vi "Determine angular axis.vi"(0 "System no.":i32=1 min=1 max=4 step=1, 2 "Axis 1":string, 3 "Axis 2":string, 5 "error in":errorcluster) -> (14 "Ang. axis out":string, 15 "Index of axis\nin Global2":i32, 16 "NC axis 1":string, 17 "NC axis 2":string, 19 "error out":errorcluster)   [LabVIEW 2020]
doc: "Determines angular axis spanned by Axis 1 and Axis 2, and NanoCube axis identifiers corresponding with Axis 1 and Axis 2."
uses:
  General command.llb/Controller names.ctl
  General command.llb/Global2 (Array).vi
panel:
  # "Determines angular axis spanned by Axis 1 and Axis 2, and \nNanoCube axis identifiers corresponding with Axis 1 and Axis 2."
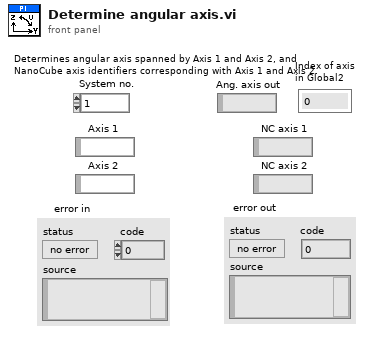
[diagram p1: front panel]
types:
  T1 = typedef "Controller names.ctl" = enum16{"None", "Analog", "C-702", "C-413", "C-414", "C-843", "C-843.PM", "C-844", "C-848", "C-865", "C-866", "C-867", "C-877", "C-880", "C-884", "C-885", "C-886", "C-887", "C-891", "E-135", "E-516", "E-517", "E-518", "E-709", "E-710", "E-712", "E-725", "E-727", "E-753", "E-754", "E-755", "E-761", "E-816", "E-861", "E-870", "E-871", "E-872", "E-873", "E-874", "F-206", "HydraPollux", "M-840", "M-850", "M-8X0", "Mercury", "Mercury_GCS", "PI_GCS2"}
  T2 = cluster{"Conn. axes":string[], "Controller name":T1}[]
  T3 = cluster{"Conn. axes":string[], "Controller name":T1}
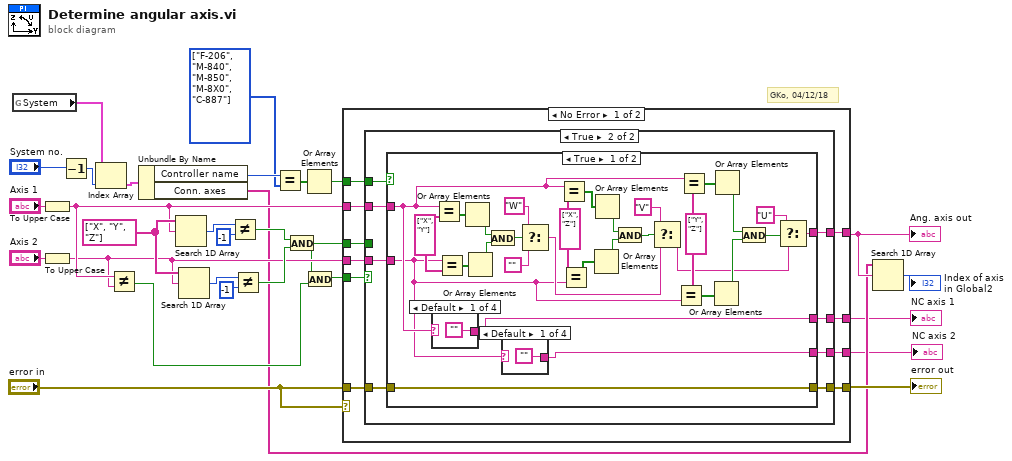
[diagram p0: block diagram]
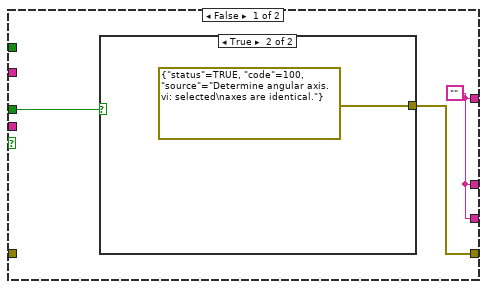
[diagram p2: hidden frame]
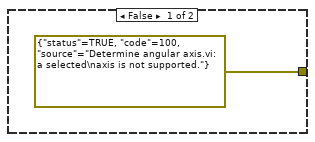
[diagram p3: hidden frame]
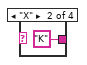
[diagram p4: hidden frame]
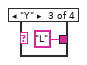
[diagram p5: hidden frame]
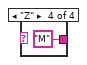
[diagram p6: hidden frame]
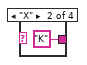
[diagram p7: hidden frame]
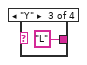
[diagram p8: hidden frame]
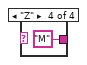
[diagram p9: hidden frame]
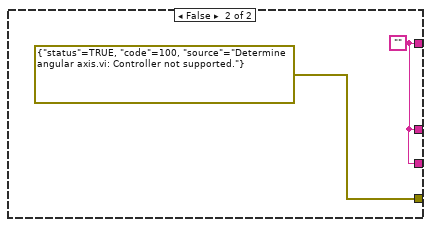
[diagram p10: hidden frame]
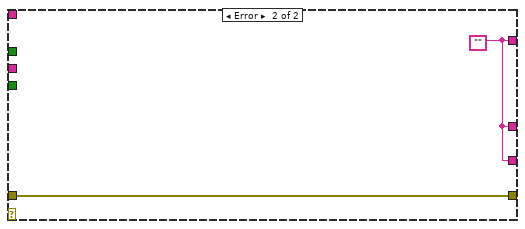
[diagram p11: hidden frame]
diagram:
  w20 = string[] ["X", "Y", "Z"]
  w23 = T1[] [enum."F-206", enum."M-840", enum."M-850", enum."M-8X0", enum."C-887"] items=["None", "Analog", "C-702", "C-413", "C-414", "C-843", "C-843.PM", "C-844", "C-848", "C-865", "C-866", "C-867", "C-877", "C-880", "C-884", "C-885", "C-886", "C-887", "C-891", "E-135", "E-516", "E-517", "E-518", "E-709", "E-710", "E-712", "E-725", "E-727", "E-753", "E-754", "E-755", "E-761", "E-816", "E-861", "E-870", "E-871", "E-872", "E-873", "E-874", "F-206", "HydraPollux", "M-840", "M-850", "M-8X0", "Mercury", "Mercury_GCS", "PI_GCS2"]
  # "GKo, 04/12/18"
  n1 = global read "Global2 (Array).vi" "System"() -> (w29:T2)
  n2 = To Upper Case(1:"Axis 1") -> (0:w12:string)
  n3 = To Upper Case(1:"Axis 2") -> (0:w11:string)
  n4 = Decrement(x="System no.") -> (x-1=w27:i32)
  n5 = Index Array(array=w29, index=w27) -> (element=w26:T3)
  n6 = Not Equal?(x=w12, y=w11) -> (x != y?=w10:bool)
  n7 = Unbundle By Name(w26) -> ("Controller name"=w24:T1, "Conn. axes"=w4:string[])
  n8 = Search 1D Array(1D array=w20, element=w12) -> (index of element=w18:i32)  [unwired: 1 out]
  n9 = Search 1D Array(1D array=w20, element=w11) -> (index of element=w17:i32)  [unwired: 1 out]
  n10 = Not Equal?(x=w18, y=-1) -> (x != y?=w16:bool)
  n11 = Not Equal?(x=w17, y=-1) -> (x != y?=w15:bool)
  n12 = Equal?(x=w24, y=w23) -> (x = y?=w22:bool[])
  n13 = And(x=w16, y=w15) -> (x .and. y?=w8:bool)
  n14 = Or Array Elements(Boolean array=w22) -> (logical OR=w21:bool)
  n15 = And(x=w8, y=w10) -> (x .and. y?=w9:bool)
  n16 = case shown="No Error" "error in" {
    tunnel: w11 -> [w39 _]
    tunnel: w12 -> [w38 _]
    tunnel: "error in" -> [w37 w94]
    tunnel: [w36 w94] -> w25
    tunnel: [w35 w93] -> w5
    tunnel: w21 -> [w34 _]
    tunnel: w9 -> [w33 _]
    tunnel: w8 -> [w32 _]
    tunnel: [w31 w93] -> w2
    tunnel: [w30 w93] -> w1
    frame No Error {
      n17 = case shown="True" w33 {
        tunnel: w39 -> [_ w52]
        tunnel: w38 -> [_ w51]
        tunnel: w37 -> [_ w50]
        tunnel: [w41 w49] -> w36
        tunnel: [w40 w48] -> w35
        tunnel: w34 -> [_ w47]
        tunnel: w32 -> [w42 _]
        tunnel: [w40 w46] -> w31
        tunnel: [w40 w45] -> w30
        frame False {
          w40 = ""
          n18 = case shown="True" w42 {
            tunnel: [errorcluster {"status"=TRUE, "code"=100, "source"="Determine angular axis.vi: a selected\naxis is not supported."} ("error out") errorcluster {"status"=TRUE, "code"=100, "source"="Determine angular axis.vi: selected\naxes are identical."} ("error out")] -> w41
            frame False {
            }
            frame True {
            }
          }
        }
        frame True {
          n19 = case shown="True" w47 {
            tunnel: w51 -> [w56 _]
            tunnel: w52 -> [w55 _]
            tunnel: [w58 w91] -> w48
            tunnel: w50 -> [w57 _]
            tunnel: [w57 errorcluster {"status"=TRUE, "code"=100, "source"="Determine angular axis.vi: Controller not supported."} ("error in")] -> w49
            tunnel: [w54 w91] -> w46
            tunnel: [w53 w91] -> w45
            frame True {
              w66 = string[] ["Y", "Z"]
              w74 = string[] ["X", "Z"]
              w82 = string[] ["X", "Y"]
              n20 = case shown="Default" w56 {
                tunnel: ["" "K" ("y") "L" ("y") "M" ("y")] -> w54
                frame Default {
                }
                frame "X" {
                }
                frame "Y" {
                }
                frame "Z" {
                }
              }
              n21 = Equal?(x=w56, y=w82) -> (x = y?=w81:bool[])
              n22 = Equal?(x=w55, y=w82) -> (x = y?=w80:bool[])
              n23 = Or Array Elements(Boolean array=w81) -> (logical OR=w79:bool)
              n24 = Or Array Elements(Boolean array=w80) -> (logical OR=w78:bool)
              n25 = And(x=w79, y=w78) -> (x .and. y?=w77:bool)
              n26 = case shown="Default" w55 {
                tunnel: ["" "K" ("y") "L" ("y") "M" ("y")] -> w53
                frame Default {
                }
                frame "X" {
                }
                frame "Y" {
                }
                frame "Z" {
                }
              }
              n27 = Select(t="W" ("y"), s=w77, f="") -> (s? t:f=w67:string)
              n28 = Equal?(x=w56, y=w74) -> (x = y?=w73:bool[])
              n29 = Equal?(x=w74, y=w55) -> (x = y?=w72:bool[])
              n30 = Or Array Elements(Boolean array=w72) -> (logical OR=w70:bool)
              n31 = Or Array Elements(Boolean array=w73) -> (logical OR=w71:bool)
              n32 = And(x=w71, y=w70) -> (x .and. y?=w69:bool)
              n33 = Select(t="V" ("y"), s=w69, f=w67) -> (s? t:f=w59:string)
              n34 = Equal?(x=w66, y=w55) -> (x = y?=w64:bool[])
              n35 = Equal?(x=w56, y=w66) -> (x = y?=w65:bool[])
              n36 = Or Array Elements(Boolean array=w64) -> (logical OR=w62:bool)
              n37 = Or Array Elements(Boolean array=w65) -> (logical OR=w63:bool)
              n38 = And(x=w63, y=w62) -> (x .and. y?=w61:bool)
              n39 = Select(t="U" ("y"), s=w61, f=w59) -> (s? t:f=w58:string)
            }
            frame False {
              w91 = ""
            }
          }
        }
      }
    }
    frame Error {
      w93 = ""
    }
  }
  "error out" <- w25
  "Ang. axis out" <- w5
  "NC axis 1" <- w2
  "NC axis 2" <- w1
  n40 = Search 1D Array(1D array=w4, element=w5) -> (index of element=→"Index of axis\nin Global2":i32)  [unwired: 1 out]
